vi "Aula_2_24022026.vi"() -> ()   [LabVIEW 2024]
panel:
  in  "Numeric 3":dbl
  in  "stop 2":bool
  out "Numeric 2":i32
  out "x*y 2":dbl
  out "°C 2":dbl(slide) scale=0.0..100.0
  in  "°F 2":dbl(slide) scale=0.0..110.0
  in  "Boolean":bool
  out "Numeric":i32
  out "x*y":dbl
  out "°C":dbl(slide) scale=0.0..100.0
  in  "°F":dbl(slide) scale=0.0..110.0
  in  "stop":bool
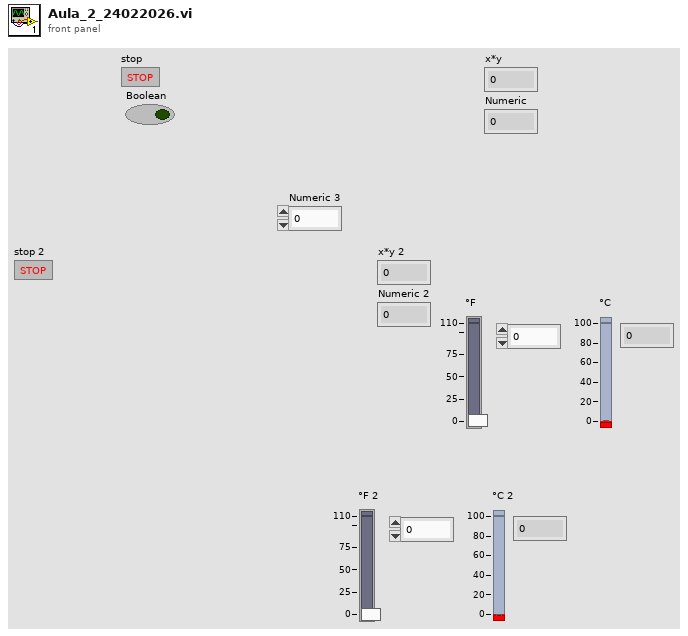
[diagram p1: front panel]
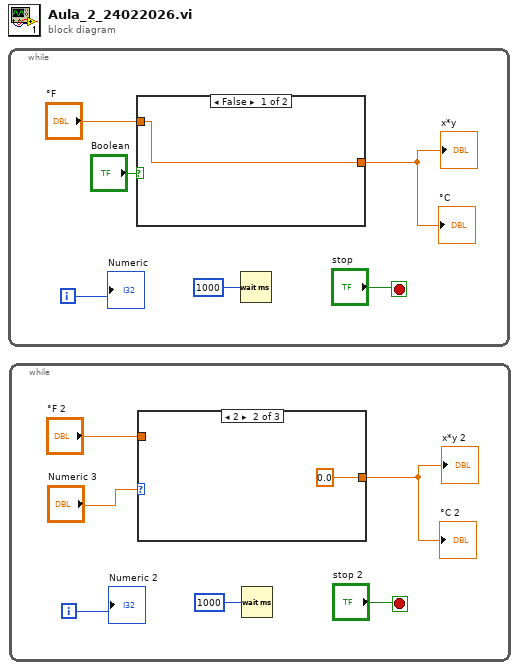
[diagram p0: block diagram]
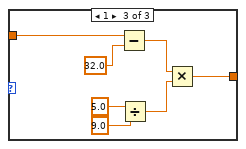
[diagram p3: hidden frame]
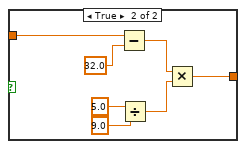
[diagram p4: hidden frame]
diagram:
  n1 = while {
    i -> [w5]
    stop <- "stop" stop-if-true
    n2 = case shown="False" "Boolean" {
      tunnel: [w7 w9] -> w4
      tunnel: "°F" -> [w7 w8]
      frame False {
      }
      frame True {
        n3 = Subtract(x=w8, y=32.0) -> (x-y=w11:dbl)
        n4 = Divide(x=5.0, y=9.0) -> (x/y=w10:dbl)
        n5 = Multiply(x=w11, y=w10) -> (x*y=w9:dbl)
      }
    }
    "x*y" <- w4
    "°C" <- w4
    n6 = Wait (ms)(milliseconds to wait=u32 1000) -> ()  [unwired: 1 out]
    "Numeric" <- w5
  }
  n7 = while {
    i -> [w19]
    stop <- "stop 2" stop-if-true
    n8 = case shown="2" "Numeric 3" {
      tunnel: [w21 0.0 ("°F 2") w24] -> w18
      tunnel: "°F 2" -> [w21 _ w23]
      frame 0, Default {
      }
      frame 2 {
      }
      frame 1 {
        n9 = Subtract(x=w23, y=32.0) -> (x-y=w26:dbl)
        n10 = Divide(x=5.0, y=9.0) -> (x/y=w25:dbl)
        n11 = Multiply(x=w26, y=w25) -> (x*y=w24:dbl)
      }
    }
    "x*y 2" <- w18
    "°C 2" <- w18
    n12 = Wait (ms)(milliseconds to wait=u32 1000) -> ()  [unwired: 1 out]
    "Numeric 2" <- w19
  }
